vi "Jpeg file pattern.vi"(0 "path":path, 3 "error in":errorcluster) -> (6 "path to JPG file":path, 9 "error out":errorcluster)   [LabVIEW 8.6]
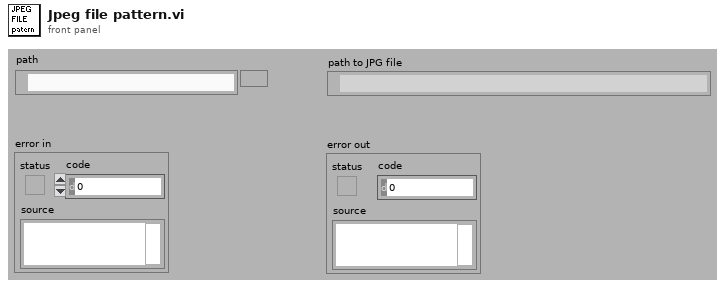
[diagram p1: front panel]
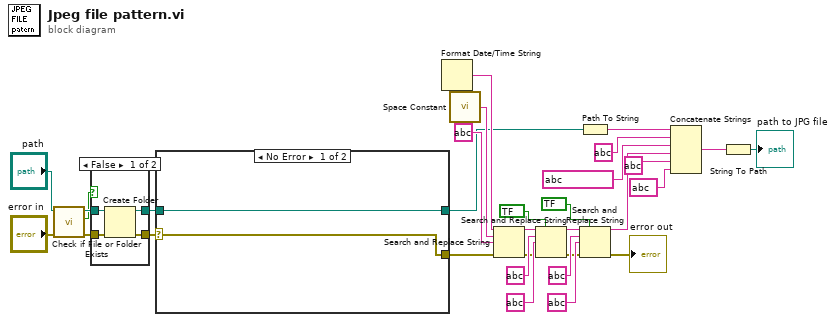
[diagram p0: block diagram]
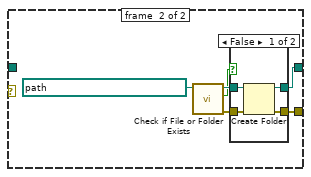
[diagram p2: hidden frame]
diagram:
  n1 = call <vilib>:"Check if File or Folder Exists.vi"("error in (no error)"="error in", "path"="path") -> ("error out"=w18:errorcluster, "file or folder exists?"=w14:bool, "dup path"=w19:path)  [unwired: 7 out]
  n2 = case shown="False" w14 {
    tunnel: [w35 w37] -> w12
    tunnel: w19 -> [w34 w37]
    tunnel: w18 -> [w33 w36]
    tunnel: [w32 w36] -> w13
    frame #0 {
      n3 = Create Folder(path (use dialog)=w34, error in=w33) -> (created path=w35:path, error out=w32:errorcluster)  [unwired: 2 out]
    }
    frame #1 {
    }
  }
  n4 = case shown="No Error" w13 {
    selector: w13 -> [w38 _]
    tunnel: w12 -> [w39 _]
    tunnel: [w39 w41] -> w11
    tunnel: [w38 w40] -> w10
    frame #0 {
    }
    frame #1 {
      n5 = call <vilib>:"Check if File or Folder Exists.vi"("path"=path ? ("path (use dialog)")) -> ("error out"=w43:errorcluster, "file or folder exists?"=w42:bool, "dup path"=w44:path)  [unwired: 1 in, 7 out]
      n6 = case shown="False" w42 {
        tunnel: [w49 w51] -> w41
        tunnel: w44 -> [w48 w51]
        tunnel: w43 -> [w47 w50]
        tunnel: [w46 w50] -> w40
        frame #0 {
          n7 = Create Folder(path (use dialog)=w48, error in=w47) -> (created path=w49:path, error out=w46:errorcluster)  [unwired: 2 out]
        }
        frame #1 {
        }
      }
    }
  }
  n8 = Format Date/Time String() -> (date/time string=w31:string)  [unwired: 3 out]
  n9 = call <vilib>:"Space Constant.vi"() -> ("String"=w30:string)
  n10 = Search and Replace String(input string=w31, search string=w30, replace string=string ? ("replace string (\"\")"), error in=w10) -> (result string=w28:string, error out=w17:errorcluster)  [unwired: 6 out]
  n11 = Search and Replace String(replace all?=bool ? ("replace all? (F)"), input string=w28, search string=string ?, replace string=string ? ("replace string (\"\")"), error in=w17) -> (result string=w21:string, error out=w16:errorcluster)  [unwired: 5 out]
  n12 = Path To String(path=w11) -> (string=w2:string)
  n13 = Search and Replace String(replace all?=bool ? ("replace all? (F)"), input string=w21, search string=string ?, replace string=string ? ("replace string (\"\")"), error in=w16) -> (result string=w4:string, error out=→"error out":errorcluster)  [unwired: 5 out]
  n14 = Concatenate Strings(w2, string ? ("string"), string ? ("string"), w4, string ? ("string"), string ? ("default name")) -> (w8:string)
  n15 = String To Path(string=w8) -> (path=→"path to JPG file":path)
